vi "Convolution.vi"() -> ()   [LabVIEW 2014]
uses:
  <vilib>/Analysis/2dsp.llb/1D Convolution (DBL).vi
  <vilib>/Analysis/NI_AALPro.lvlib
panel:
  out "DTFT{x(n)*y(n)}":cluster{"-pi to pi":dbl[], "DTFT op":dbl[]}(graph)
  out "X(w).Y(w)":cluster{"-pi to pi":dbl[], dbl[]}(graph)
  in  "Boolean":bool
  out "DTFT{x(n)*y(n)}":cdb[](array[numeric])
  out "X(w).Y(w)":cdb[](array[numeric])
  out "x(n)*y(n)":dbl[](array[numeric])
  in  "y(n)":dbl[](array[numeric])
  in  "x(n)":dbl[](array[numeric])
  # "if \nDTFT{x(n)}  ---->  X(w)\nDTFT{y(n)}  ----->  Y(w)\nthen          DTFT\nx(n)*y(n)  ----->  X(w).Y(w)"
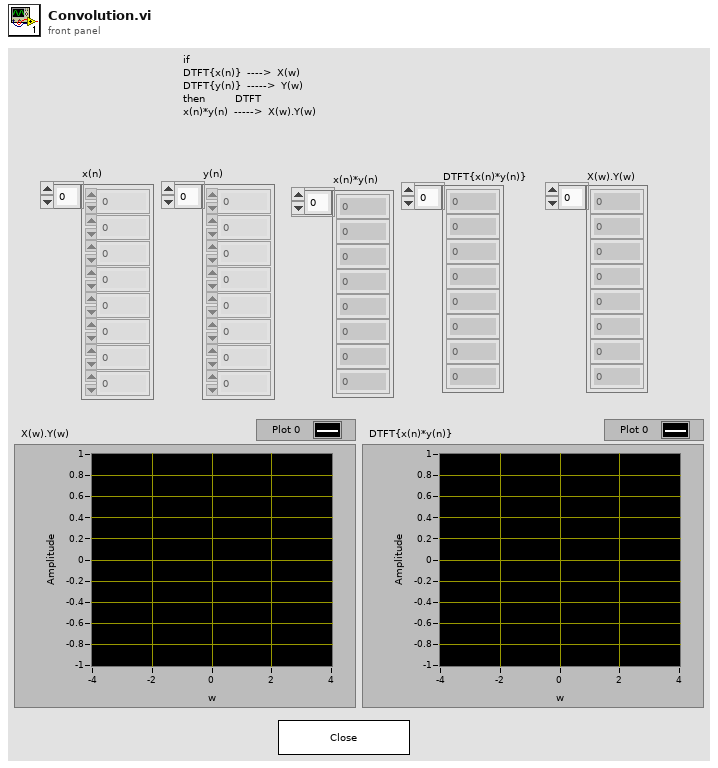
[diagram p1: front panel]
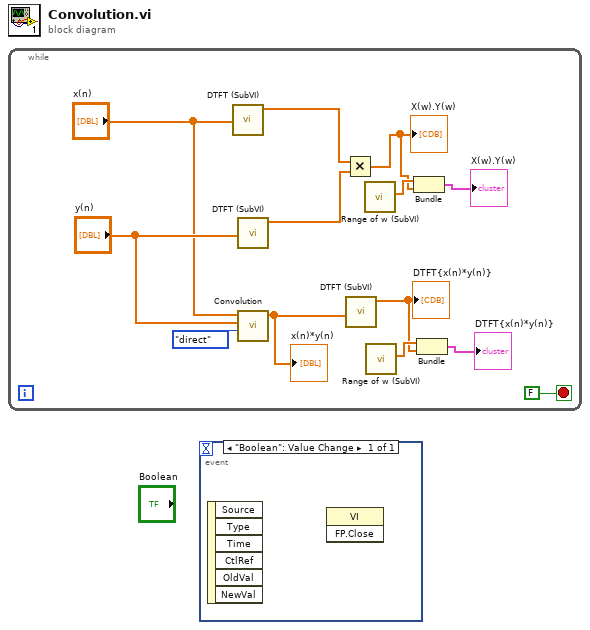
[diagram p0: block diagram]
diagram:
  n1 = while {
    stop <- FALSE stop-if-true
    n2 = call "DTFT (SubVI).vi"("ip array"="x(n)") -> ("DTFT op"=w9:cdb[])  [unwired: 9 in, 1 out]
    n3 = call "DTFT (SubVI).vi"("ip array"="y(n)") -> ("DTFT op"=w8:cdb[])  [unwired: 9 in, 1 out]
    n4 = call-poly <vilib>:"Convolution.vi"("algorithm"=enum32{"direct", "frequency domain"}."direct", "Y"="y(n)", "X"="x(n)") -> ("X * Y"=w10:dbl[])  [unwired: 7 in, 1 out]
    "x(n)*y(n)" <- w10
    n5 = Multiply(x=w9, y=w8) -> (x*y=w4:cdb[])
    "X(w).Y(w)" <- w4
    n6 = call "DTFT (SubVI).vi"("ip array"=w10) -> ("DTFT op"=w3:cdb[])  [unwired: 9 in, 1 out]
    "DTFT{x(n)*y(n)}" <- w3
    n7 = call "Range of w (SubVI).vi"() -> ("-pi to pi"=w5:dbl[])  [unwired: 11 in]
    n8 = call "Range of w (SubVI).vi"() -> ("-pi to pi"=w6:dbl[])  [unwired: 11 in]
    n9 = Bundle("-pi to pi"=w5, w4) -> (→"X(w).Y(w)":cluster{"-pi to pi":dbl[], cdb[]})  [unwired: 1 in]
    n10 = Bundle("-pi to pi"=w6, "DTFT op"=w3) -> (→"DTFT{x(n)*y(n)}":cluster{"-pi to pi":dbl[], "DTFT op":cdb[]})  [unwired: 1 in]
  }
  n11 = event shown="[0] \"Boolean\": Value Change" {
    selector: _ -> [_]
    dyn-events: _ -> [_]
    timeout: _ -> [_]
    event "Boolean": Value Change {
      n12 = event-data() -> ()  [unwired: 1 in, 6 out]
      n13 = invoke class="VI" method="FP.Close"() -> ()  [unwired: 3 in, 3 out]
    }
  }
